vi "PM-close.vi"(8 "error out":errorcluster, 11 "init_cluster":T1) -> (0 "error out out":errorcluster)   [LabVIEW 2018]
uses:
  PM-init-data_cluster.ctl
  PM-init-user_events.ctl
  PM-common-heartrate_data.ctl
  PM-common-peak-detect_settings.ctl
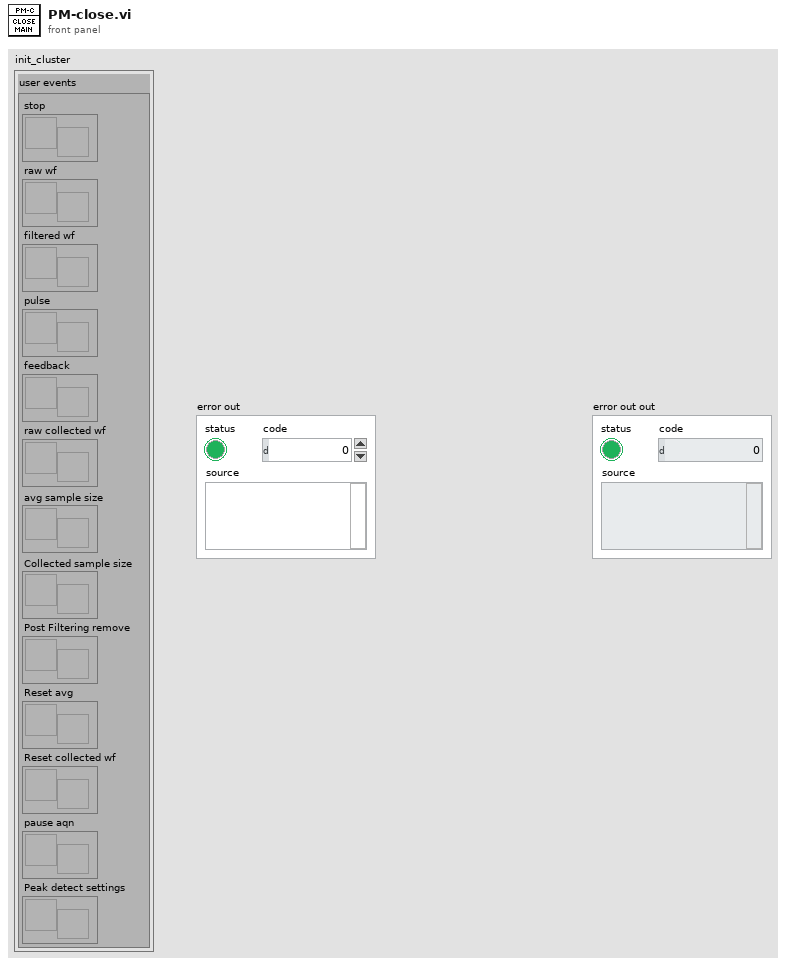
[diagram p1: front panel]
types:
  T1 = typedef "PM-init-data_cluster.ctl" = cluster{"user events":T2}
  T2 = typedef "PM-init-user_events.ctl" = cluster{"stop":refnum<user-event>, "raw wf":refnum<user-event>, "filtered wf":refnum<user-event>, "pulse":refnum<user-event>, "feedback":refnum<user-event>, "raw collected wf":refnum<user-event>, "avg sample size":refnum<user-event>, "Collected sample size":refnum<user-event>, "Post Filtering remove":refnum<user-event>, "Reset avg":refnum<user-event>, "Reset collected wf":refnum<user-event>, "pause aqn":refnum<user-event>, "Peak detect settings":refnum<user-event>}
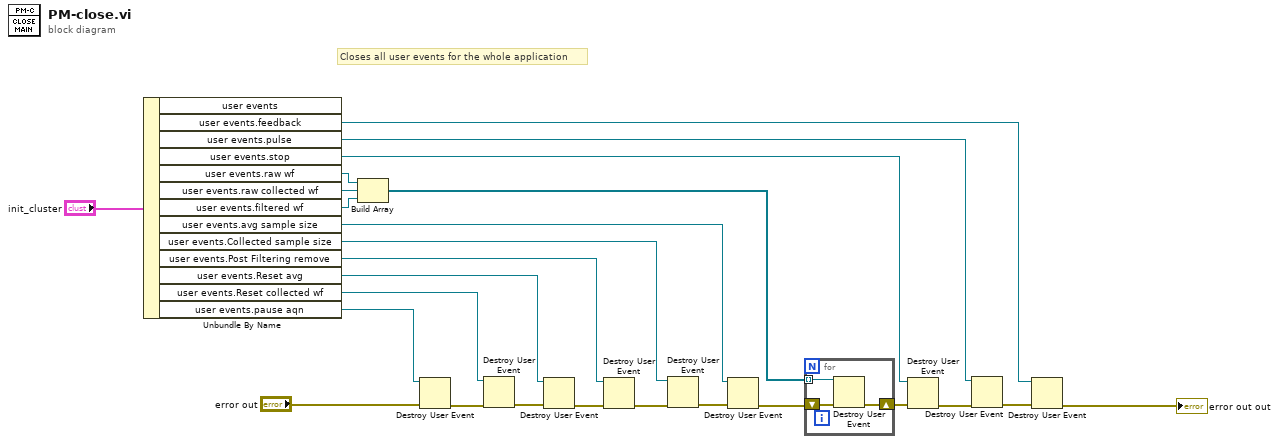
[diagram p0: block diagram]
diagram:
  # "Closes all user events for the whole application"
  n1 = Unbundle By Name("init_cluster") -> ("user events.feedback"=w14:refnum<user-event>, "user events.pulse"=w15:refnum<user-event>, "user events.stop"=w16:refnum<user-event>, "user events.raw wf"=w20:refnum<user-event>, "user events.raw collected wf"=w19:refnum<user-event>, "user events.filtered wf"=w18:refnum<user-event>, "user events.avg sample size"=w11:refnum<user-event>, "user events.Collected sample size"=w10:refnum<user-event>, "user events.Post Filtering remove"=w9:refnum<user-event>, "user events.Reset avg"=w5:refnum<user-event>, "user events.Reset collected wf"=w4:refnum<user-event>, "user events.pause aqn"=w3:refnum<user-event>)  [unwired: 1 out]
  n2 = Build Array(w20, w19, w18) -> (w17:refnum<user-event>[])
  n3 = Destroy User Event(user event=w3, error in="error out") -> (error out=w7:errorcluster)
  n4 = Destroy User Event(user event=w4, error in=w7) -> (error out=w8:errorcluster)
  n5 = Destroy User Event(user event=w5, error in=w8) -> (error out=w6:errorcluster)
  n6 = Destroy User Event(user event=w9, error in=w6) -> (error out=w13:errorcluster)
  n7 = Destroy User Event(user event=w10, error in=w13) -> (error out=w12:errorcluster)
  n8 = Destroy User Event(user event=w11, error in=w12) -> (error out=w1:errorcluster)
  n9 = for {
    shift-right: [w27] -> w22
    shift-left: w1 -> [w28]
    tunnel: w17 -> [w26] mode=indexing
    n10 = Destroy User Event(user event=w26, error in=w28) -> (error out=w27:errorcluster)
  }
  n11 = Destroy User Event(user event=w16, error in=w22) -> (error out=w21:errorcluster)
  n12 = Destroy User Event(user event=w15, error in=w21) -> (error out=w24:errorcluster)
  n13 = Destroy User Event(user event=w14, error in=w24) -> (error out=→"error out out":errorcluster)
